vi "Replace dt DBL.vi"(10 "dt":dbl, 11 "Waveform in":waveform(dbl)) -> (3 "Waveform out":waveform(dbl))   [LabVIEW 2015]
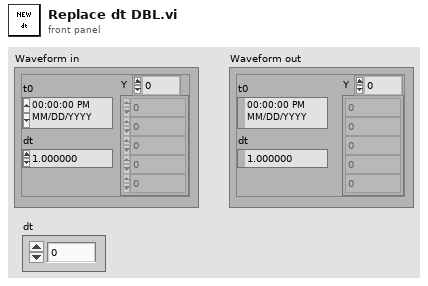
[diagram p1: front panel]
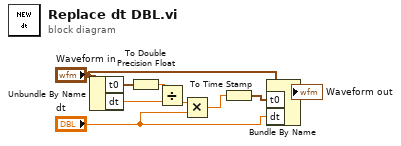
[diagram p0: block diagram]
diagram:
  n1 = Unbundle By Name("Waveform in") -> ("t0"=w3:timestamp, "dt"=w5:dbl)
  n2 = To Double Precision Float(number=w3) -> (double precision float=w4:dbl)
  n3 = Divide(x=w4, y=w5) -> (x/y=w6:dbl)
  n4 = Multiply(x=w6, y="dt") -> (x*y=w7:dbl)
  n5 = To Time Stamp(1:w7) -> (0:w8:timestamp)
  n6 = Bundle By Name(cluster="Waveform in", "t0"=w8, "dt"="dt") -> (→"Waveform out":waveform(dbl))
